vi "Read Temperatures DBL.vi"(8 "error in":errorcluster, 10 "Source":string, 11 "IRead Temperatures Multichannel in":refnum<class "IRead Temperature Multichannel.lvclass">) -> (0 "error out":errorcluster, 1 "Timestamps":timestamp[](array[timestamp]) format="%<%x %.3X>T", 2 "Temperatures":dbl[](array[numeric]), 3 "IRead Temperatures Multichannel out":refnum<class "IRead Temperature Multichannel.lvclass">)   [LabVIEW 2024, in "IRead Temperature Multichannel.lvclass"]
uses:
  IRead Temperature Multichannel.lvclass
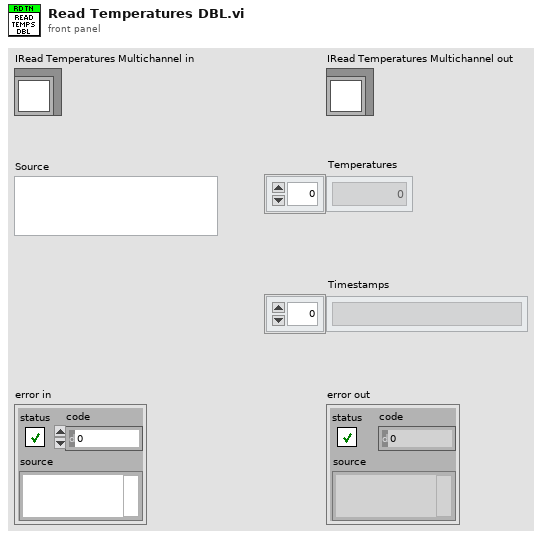
[diagram p1: front panel]
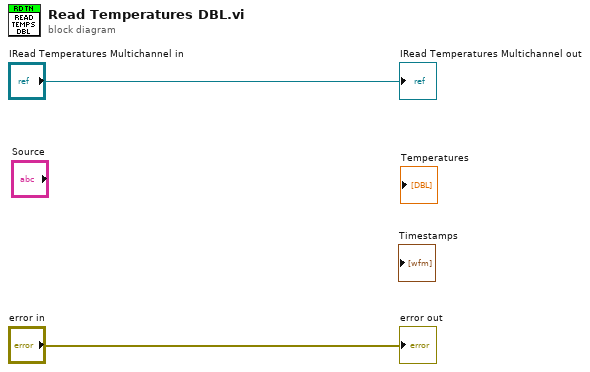
[diagram p0: block diagram]
diagram:
  "error out" <- "error in"
  "IRead Temperatures Multichannel out" <- "IRead Temperatures Multichannel in"
